vi "DAQ.GenerateWaveform.Override.vi"(8 "error in (no error)":errorcluster, 11 "DAQ in":refnum<class "DAQ.lvclass">) -> (0 "error out":errorcluster, 2 "Waveforms":waveform(dbl)[](array[waveform]), 3 "DAQ out":refnum<class "DAQ.lvclass">)   [LabVIEW 2016, in "DAQ.lvclass"]
uses:
  DAQ.lvclass
  <vilib>/measure/NI_MABase.lvlib
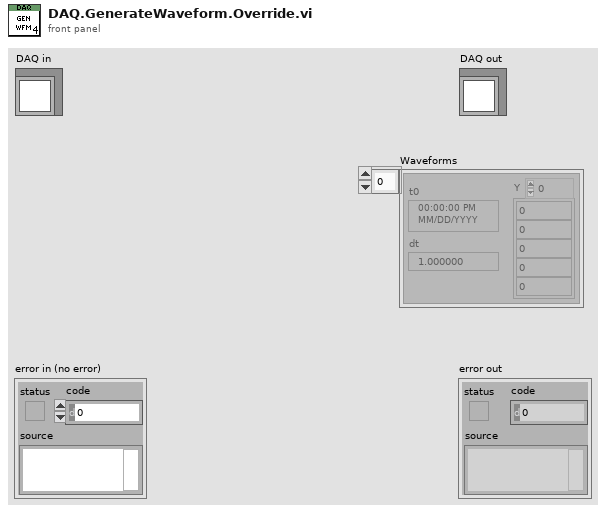
[diagram p1: front panel]
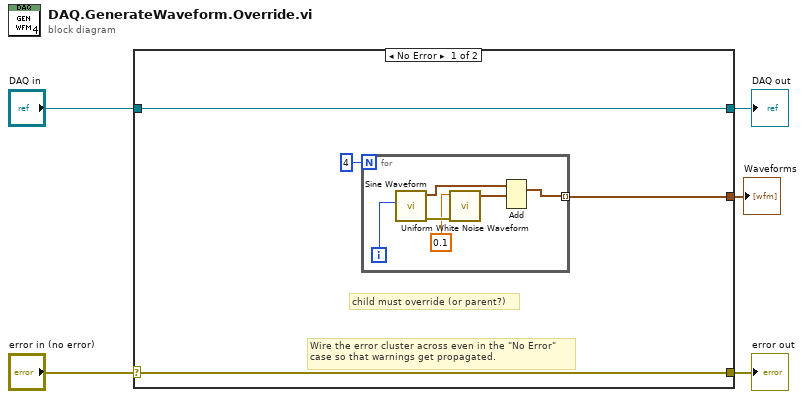
[diagram p0: block diagram]
diagram:
  n1 = case shown="No Error" "error in (no error)" {
    selector: "error in (no error)" -> [w8 w17]
    tunnel: [w8 w17] -> w4
    tunnel: [w9 w16] -> w2
    tunnel: "DAQ in" -> [w9 w16]
    tunnel: [w6 _] -> w1
    frame No Error {
      # "child must override (or parent?)"
      # "Wire the error cluster across even in the \"No Error\"\ncase so that warnings get propagated."
      n2 = for {
        N: 4 -> [_]
        tunnel: [w11] -> w6 mode=indexing
        i -> [w15]
        n3 = call <vilib>:"Sine Waveform.vi"("amplitude"=w15) -> ("error out"=w14:errorcluster, "signal out"=w12:waveform(dbl))  [unwired: 9 in]
        n4 = call <vilib>:"Uniform White Noise Waveform.vi"("error in (no error)"=w14, "amplitude"=0.1) -> ("signal out"=w13:waveform(dbl))  [unwired: 8 in, 1 out]
        n5 = Add(1:w13, 2:w12) -> (0:w11:waveform(dbl))  [unwired: 1 in, 1 out]
      }
    }
    frame Error {
    }
  }
  "error out" <- w4
  "DAQ out" <- w2
  "Waveforms" <- w1
